vi "RES2 Time.vi"() -> ()   [LabVIEW 2015]
panel:
  out "output array":dbl[](array[numeric])
  out "Waveform Graph 3":dbl[](graph)
  out "Waveform Graph 2":dbl[](graph)
  out "error out":errorcluster={"status"=TRUE, "code"=-1074126836, "source"="niSwitch Connect Channels.vi<ERR>Driver Status:  (Hex 0xBFFA200C) An explicit connection between the channels already exists.\n\nChannel Names: ch0, com0\nDevice: 2503_PXI1Slot14\n\nStatus Code: -200179\n\n "}
  out "x-y":u32
  in  "variable":T1={"resource1"={"2503"="2503_PXI1Slot3", "4070"="4070_PXI1Slot2", "2530"=["2530_PXI1Slot4", "2530_PXI1Slot5", "2530_PXI1Slo6", "2530_PXI1Slot7", "2530_PXI1Slot8", "2530_PXI1Slot9", "2530_PXI1Slot10"]}, "resource2"={"2503"="2503_PXI1Slot12", "4070"="4070_PXI1Slot11", "2530"=["2530_PXI1Slot13", "2530_PXI1Slot14", "2530_PXI1Slot15"]}, "resource3"={"2530"="2530_PXI1Slot17", "4070"="4070_PXI1Slot16"}, "error in"={"status"=FALSE, "code"=0, "source"=""}} {"error in"."code" format="%.0x"}
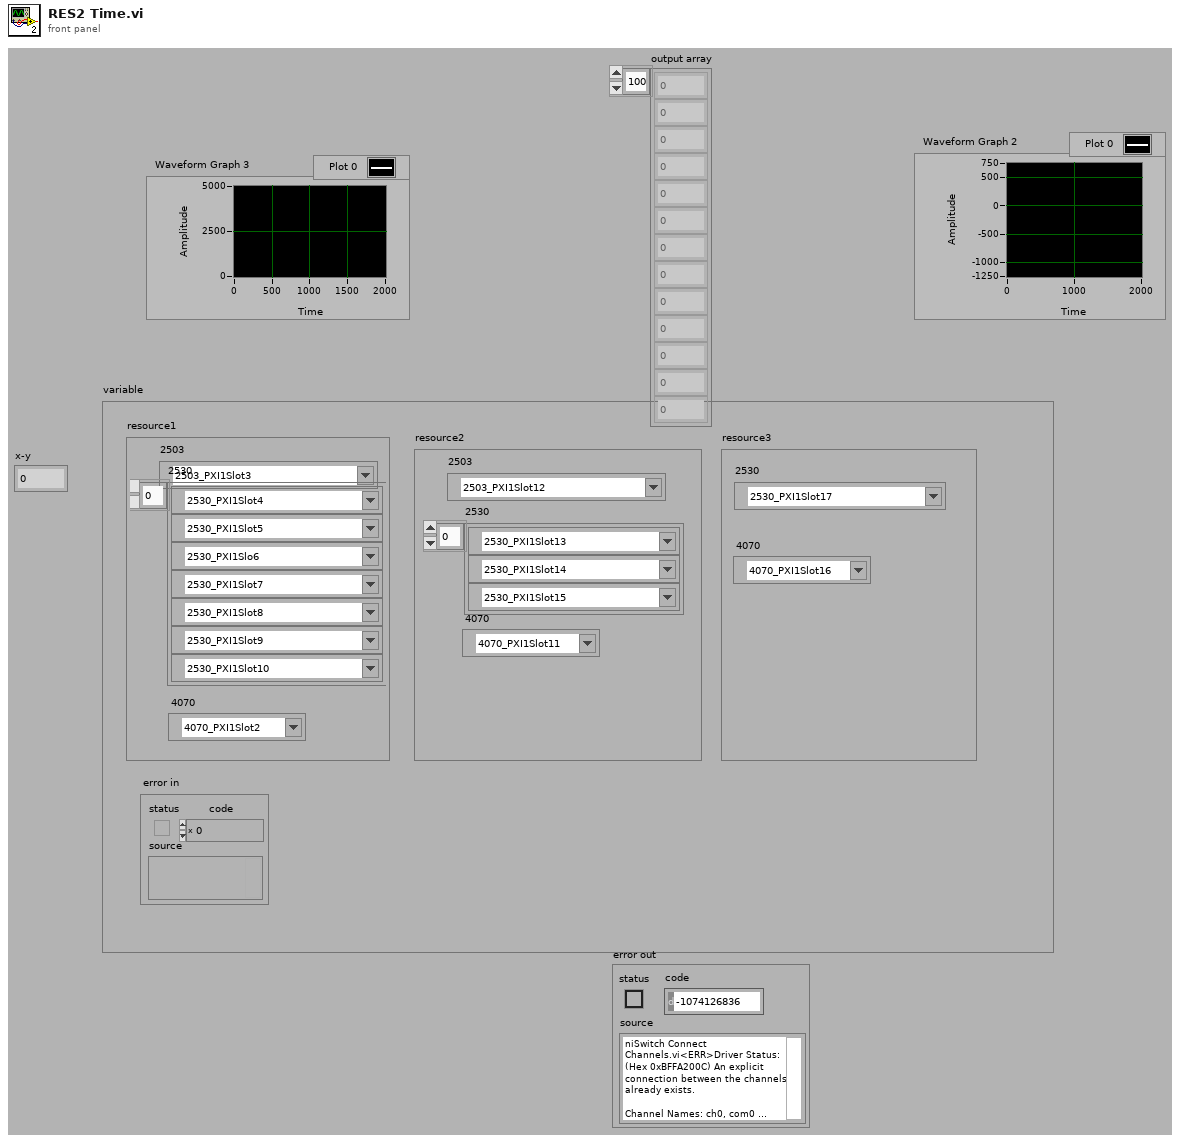
[diagram p1: front panel]
types:
  T1 = cluster{"resource1":cluster{"2503":refnum<k15>, "4070":refnum<k15>, "2530":refnum<k15>[]}, "resource2":cluster{"2503":refnum<k15>, "4070":refnum<k15>, "2530":refnum<k15>[]}, "resource3":cluster{"2530":refnum<k15>, "4070":refnum<k15>}, "error in":errorcluster}
  T2 = cluster{"2503":refnum<k15>, "4070":refnum<k15>, "2530":refnum<k15>[]}
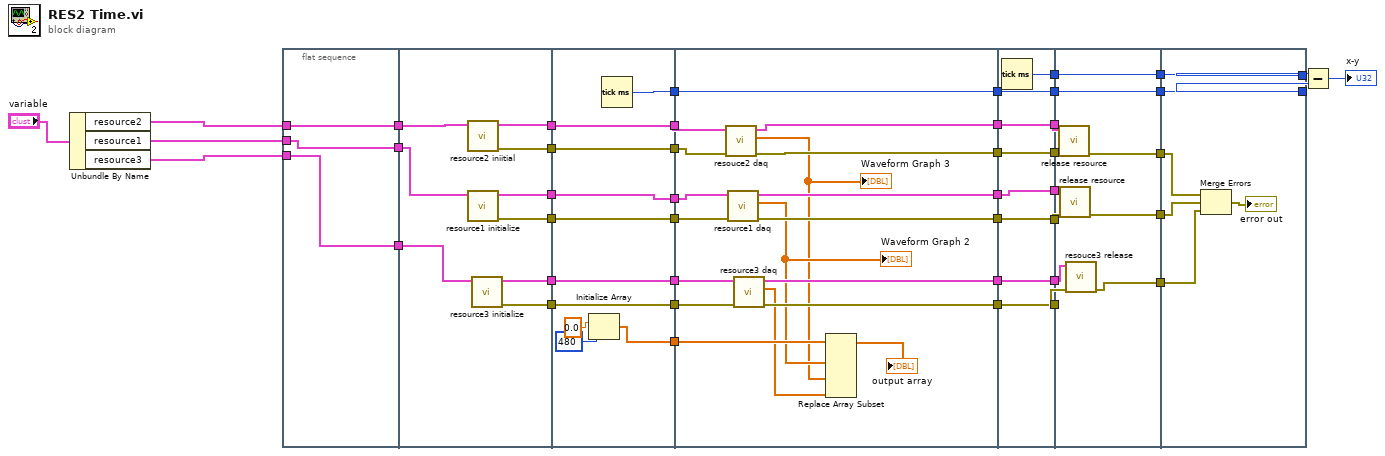
[diagram p0: block diagram]
diagram:
  n1 = Unbundle By Name("variable") -> ("resource2"=w43:T2, "resource1"=w23:T2, "resource3"=w11:cluster{"2530":refnum<k15>, "4070":refnum<k15>})
  n2 = flat-sequence {
    tunnel: w43 -> [w47]
    tunnel: [w47] -> w41
    tunnel: w23 -> [w46]
    tunnel: [w46] -> w22
    tunnel: [w45] -> w12
    tunnel: w11 -> [w45]
    tunnel: w41 -> [w56]
    tunnel: [w55] -> w40
    tunnel: [w54] -> w38
    tunnel: w22 -> [w53]
    tunnel: [w52] -> w21
    tunnel: [w51] -> w17
    tunnel: w12 -> [w50]
    tunnel: [w49] -> w9
    tunnel: [w48] -> w4
    tunnel: w40 -> [w66]
    tunnel: [w66] -> w39
    tunnel: w38 -> [w65]
    tunnel: [w65] -> w37
    tunnel: [w64] -> w36
    tunnel: w21 -> [w63]
    tunnel: [w63] -> w20
    tunnel: w17 -> [w62]
    tunnel: [w62] -> w16
    tunnel: [w61] -> w10
    tunnel: w9 -> [w61]
    tunnel: [w60] -> w5
    tunnel: w4 -> [w60]
    tunnel: [w57] -> w1
    tunnel: w39 -> [w84]
    tunnel: w37 -> [w83]
    tunnel: w36 -> [w82]
    tunnel: [w82] -> w33
    tunnel: [w81] -> w31
    tunnel: [w80] -> w29
    tunnel: w20 -> [w79]
    tunnel: [w78] -> w19
    tunnel: w16 -> [w77]
    tunnel: [w76] -> w15
    tunnel: w10 -> [w75]
    tunnel: [w74] -> w7
    tunnel: w5 -> [w73]
    tunnel: [w72] -> w2
    tunnel: w1 -> [w71]
    tunnel: w33 -> [w92]
    tunnel: [w92] -> w32
    tunnel: w31 -> [w91]
    tunnel: [w91] -> w30
    tunnel: w29 -> [w90]
    tunnel: [w90] -> w28
    tunnel: [w89] -> w27
    tunnel: w19 -> [w88]
    tunnel: [w88] -> w18
    tunnel: w15 -> [w87]
    tunnel: [w87] -> w14
    tunnel: [w86] -> w8
    tunnel: w7 -> [w86]
    tunnel: [w85] -> w3
    tunnel: w2 -> [w85]
    tunnel: [w103] -> w35
    tunnel: w32 -> [w103]
    tunnel: w30 -> [w102]
    tunnel: w28 -> [w101]
    tunnel: [w100] -> w34
    tunnel: w27 -> [w99]
    tunnel: [w99] -> w26
    tunnel: w18 -> [w98]
    tunnel: w14 -> [w97]
    tunnel: [w96] -> w13
    tunnel: w8 -> [w95]
    tunnel: [w94] -> w6
    tunnel: w3 -> [w93]
    tunnel: [w109] -> w24
    tunnel: w35 -> [w109]
    tunnel: w34 -> [w107]
    tunnel: w26 -> [w108]
    tunnel: [w108] -> w25
    tunnel: w13 -> [w106]
    tunnel: w6 -> [w105]
    frame #0 {
    }
    frame #1 {
      n3 = call "resource2 iniitial.vi"("resource1"=w56) -> ("error out"=w54:errorcluster, "resource1 out"=w55:T2)  [unwired: 9 in]
      n4 = call "resource1 initialize.vi"("resource1"=w53) -> ("error out"=w51:errorcluster, "resource1 out"=w52:T2)  [unwired: 9 in]
      n5 = call "resource3 initialize.vi"("resource3"=w50) -> ("error out"=w48:errorcluster, "output cluster"=w49:cluster{"2530":refnum<k15>, "4070":refnum<k15>})  [unwired: 9 in]
    }
    frame #2 {
      n6 = Initialize Array(0.0 ("element"), 480 ("dimension size")) -> (w57:dbl[])
      n7 = Tick Count (ms)() -> (millisecond timer value=w64:u32)
    }
    frame #3 {
      n8 = call "resouce2 daq.vi"("error in"=w83, "resouce2"=w84) -> ("error out"=w80:errorcluster, "value"=w68:dbl[], "resouce2 out"=w81:T2)  [unwired: 7 in]
      "Waveform Graph 3" <- w68
      n9 = call "resource1 daq.vi"("error in"=w77, "resource1"=w79) -> ("error out"=w76:errorcluster, "value"=w69:dbl[], "resoure1 out"=w78:T2)  [unwired: 7 in]
      "Waveform Graph 2" <- w69
      n10 = call "resource3 daq.vi"("error in"=w73, "resource3"=w75) -> ("error out"=w72:errorcluster, "Value"=w70:dbl[], "output cluster"=w74:cluster{"2530":refnum<k15>, "4070":refnum<k15>})  [unwired: 7 in]
      n11 = Replace Array Subset(array=w71, new element #1=w69, new element #2=w68, new element #3=w70) -> (→"output array":dbl[])  [unwired: 3 in]
    }
    frame #4 {
      n12 = Tick Count (ms)() -> (millisecond timer value=w89:u32)
    }
    frame #5 {
      n13 = call "release resource.vi"("error in"=w101, "resource"=w102) -> ("error out"=w100:errorcluster)  [unwired: 9 in]
      n14 = call "release resource.vi"("error in"=w97, "resource"=w98) -> ("error out"=w96:errorcluster)  [unwired: 9 in]
      n15 = call "resouce3 release.vi"("error in"=w93, "resource3"=w95) -> ("error out"=w94:errorcluster)  [unwired: 9 in]
    }
    frame #6 {
      n16 = Merge Errors(w107, w106, w105) -> (→"error out":errorcluster)
    }
  }
  n17 = Subtract(x=w25, y=w24) -> (x-y=→"x-y":u32)
